vi "界面UI.vi"() -> ()   [LabVIEW 2016, in "科盛超标留样.lvlib"]
uses:
  <vilib>/Utility/miscctls.llb/LVPointTypeDef.ctl
  <vilib>/Utility/config.llb/NI_LVConfig.lvlib
  <vilib>/ptbypt/NI_PtbyPt.lvlib
panel:
  in  "参数设置":bool
  out "留样模式":T1(ring)
  out "仪器时间":timestamp format="%<%Y/%m/%d %H:%M:%S>T"
  out "采样器状态":enum16{"待机", "运行中"}(ring)
  in  "停止流程":bool
  in  "启动流程":bool
  out "流程中":bool
  out "留样等待时间/s":dbl
  out "供样等待时间/s":dbl
  out "采样等待时间/s":dbl
  out "留样完成":bool
  out "采样完成":bool
  out "开关量3状态":T2
  out "开关量2状态":T3
  out "开关量1状态":T4
  out "供样完成":bool
  in  "返回":bool
  in  "查看记录":bool
  out "查询系统状态":T5
  in  "留样命令":bool
  in  "供样命令":bool
  in  "触发采样":bool
  in  "远程取样":bool
  in  "复位指令":bool
  out "VISA resource name":refnum<visa-resource-name>="COM2" caption="VISA资源名称"
  out "读取缓冲区":string
  out "source":string
  out "通讯":bool
  # "启动顺序：\n①先触发采样将水样取到A、B桶\n②然后仪器开始测试时发送供样命令此时供应到分析仪\n③如果超标发送留样命令，如果在默认60分钟(可设置)后都没有接受到超标留\n样指令则自动排空。按不同的采样方式发送不同的通信字符串。在一次采样未结束前不要发送下一个采样指令。"
  # "采样：将水样取到A、B桶的过程；\n供样：将水样从A、B桶供应到分析仪的过程；\n留样：将水样从A、B桶保存到采样瓶的过程。"
  # "科盛超标留样"
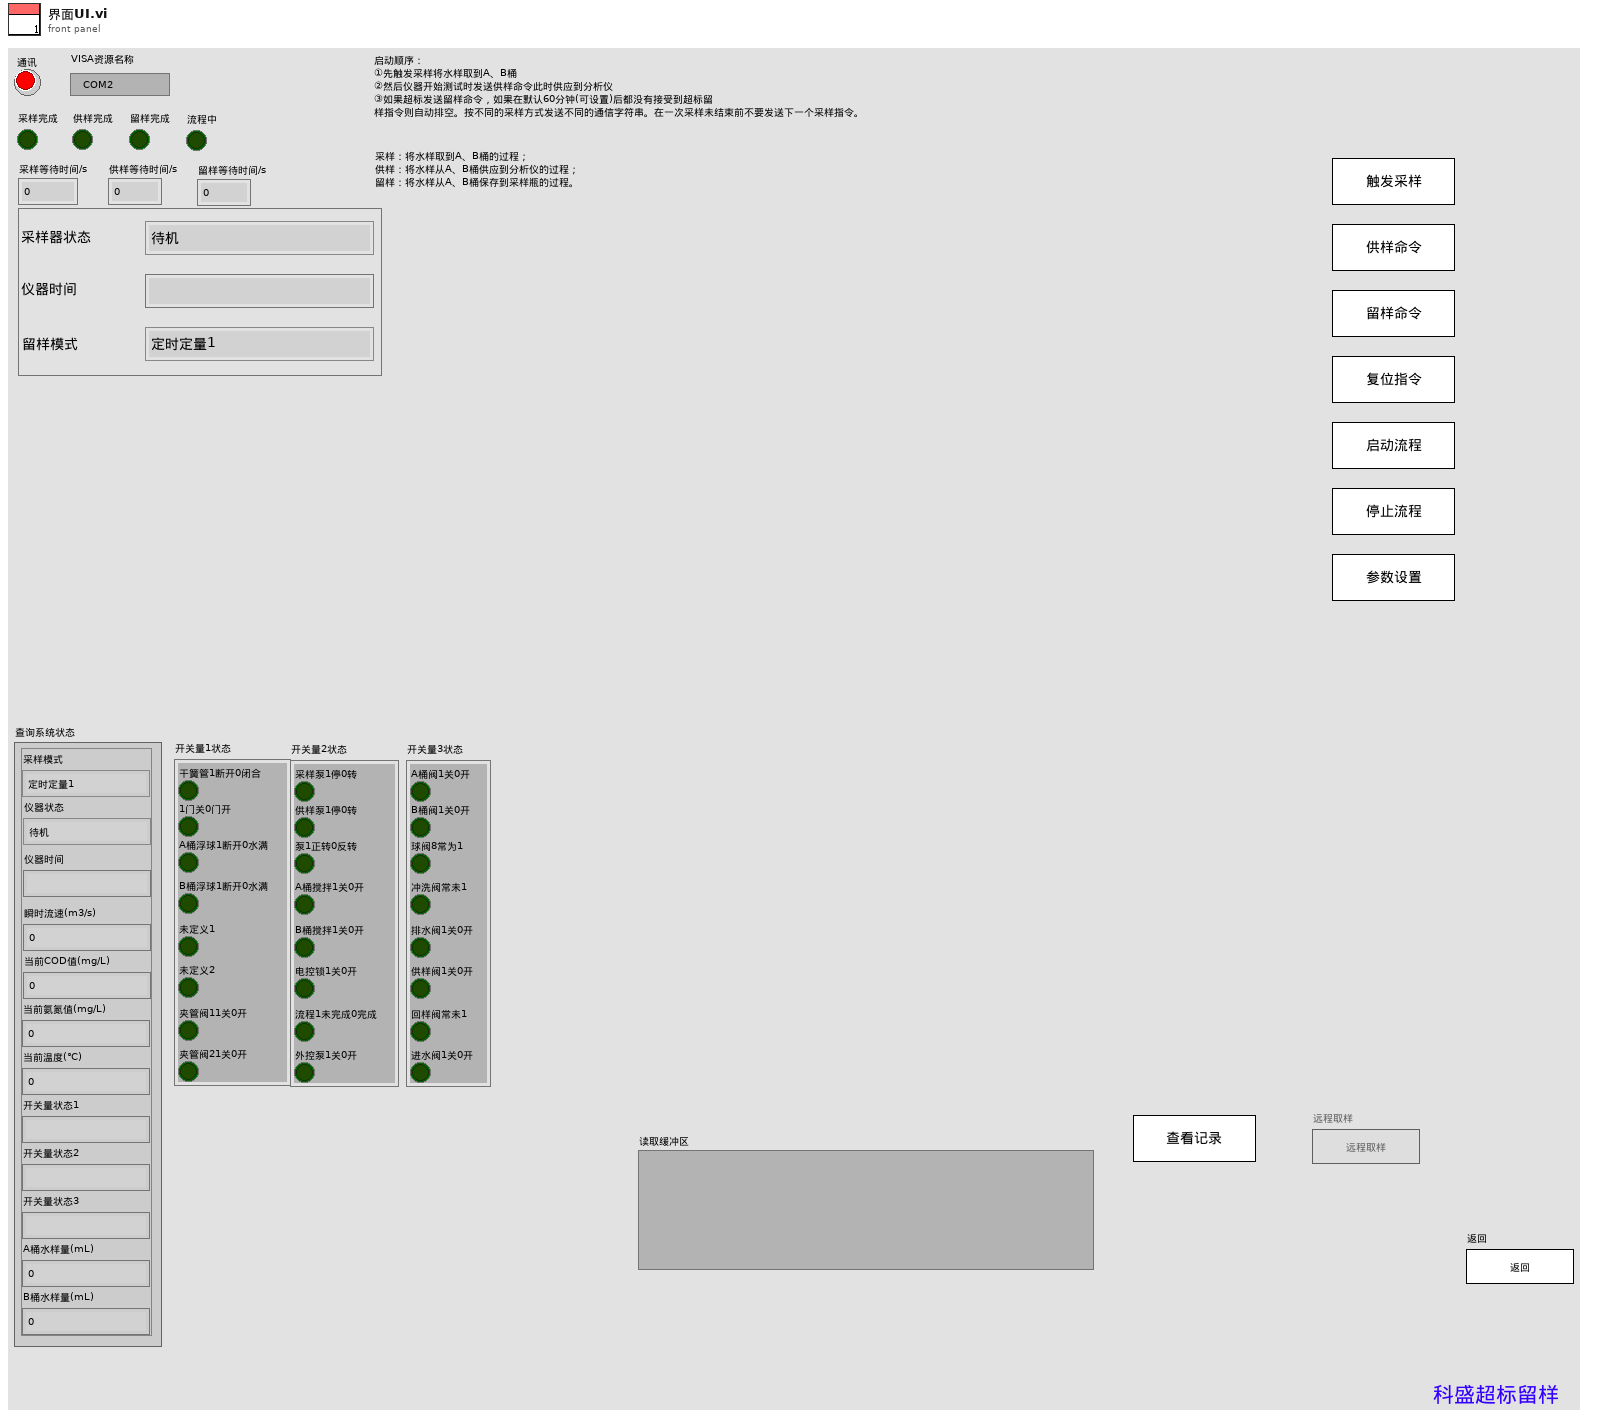
[diagram p1: front panel]
types:
  T1 = enum16{"定时定量1", "定时定量2", "定流定量", "定时比例", "同步留样", "超标留样", "触发采样", "定时采样1", "定流供样", "定时采样2", "远程取样", "手动取样", "流量跟踪"}
  T2 = cluster{"A桶阀1关0开":bool, "B桶阀1关0开":bool, "球阀8常为1":bool, "冲洗阀常未1":bool, "排水阀1关0开":bool, "供样阀1关0开":bool, "回样阀常未1":bool, "进水阀1关0开":bool}
  T3 = cluster{"采样泵1停0转":bool, "供样泵1停0转":bool, "泵1正转0反转":bool, "A桶搅拌1关0开":bool, "B桶搅拌1关0开":bool, "电控锁1关0开":bool, "流程1未完成0完成":bool, "外控泵1关0开":bool}
  T4 = cluster{"干簧管1断开0闭合":bool, "1门关0门开":bool, "A桶浮球1断开0水满":bool, "B桶浮球1断开0水满":bool, "未定义1":bool, "未定义2":bool, "夹管阀11关0开":bool, "夹管阀21关0开":bool}
  T5 = cluster{"采样模式":enum16{"定时定量1", "定时定量2", "定流定量", "定时比例", "同步留样", "超标留样", "触发采样", "定时采样1", "定流供样", "定时采样2", "远程取样", "手动取样", "流量跟踪"}, "仪器状态":enum16{"待机", "运行中"}, "仪器时间":string, "瞬时流速(m3/s)":dbl, "当前COD值(mg/L)":dbl, "当前氨氮值(mg/L)":dbl, "当前温度(℃)":dbl, "开关量状态1":string, "开关量状态2":string, "开关量状态3":string, "A桶水样量(mL)":dbl, "B桶水样量(mL)":dbl}
  T6 = cluster{"枚举":enum16{"open", "read", "write", "close"}, "写入字符串":string, "解析字符串":string}
  T7 = cluster{"STEP":enum16{"open", "read", "write", "close"}, "写入缓冲区":string}
  T8 = enum16{"触发采样", "供样命令", "留样命令", "远程取样", "复位指令", "查询采样记录", "查询瓶记录", "查询系统状态"}
  T9 = typedef "LVPointTypeDef.ctl" = cluster{"Horizontal":i16, "Vertical":i16}
  T10 = typedef "NI_LVConfig.lvlib/Config Data RefNum.ctl" = refnum<k1>
  T11 = enum32{"Bad", "Idle", "Run top level", "Running"}
  T12 = cluster{"命令":string, "data":cluster{"starting address":u16, "coil values":bool[]}}
  T13 = enum8{"Enabled", "Disabled", "Disabled and Grayed Out"}
  T14 = cluster{"[0]":bool, "[1]":bool, "[2]":bool, "[3]":bool, "[4]":bool, "[5]":bool, "[6]":bool, "[7]":bool}
  T15 = cluster{"采样时间":string, "采样模式":enum16{"定时定量1", "定时定量2", "定流定量", "定时比例", "同步留样", "超标留样", "触发采样", "定时采样1", "定流供样", "定时采样2", "远程取样", "手动取样", "流量跟踪"}, "采样瓶":string, "混采n次，设定混采n次":string, "当前采样量(ml)":dbl, "当前瓶内总水样量(ml)":dbl, "当前瓶号平行样，设定平行样":string}[]
  T16 = cluster{"瓶1采样量(ml)":dbl, "瓶2采样量(ml)":dbl, "瓶3采样量(ml)":dbl, "瓶4采样量(ml)":dbl, "瓶5采样量(ml)":dbl, "瓶6采样量(ml)":dbl, "瓶7采样量(ml)":dbl, "瓶8采样量(ml)":dbl, "瓶9采样量(ml)":dbl, "瓶10采样量(ml)":dbl, "瓶11采样量(ml)":dbl, "瓶12采样量(ml)":dbl, "瓶13采样量(ml)":dbl, "瓶14采样量(ml)":dbl, "瓶15采样量(ml)":dbl, "瓶16采样量(ml)":dbl, "瓶17采样量(ml)":dbl, "瓶18采样量(ml)":dbl, "瓶19采样量(ml)":dbl, "瓶20采样量(ml)":dbl, "瓶21采样量(ml)":dbl, "瓶22采样量(ml)":dbl, "瓶23采样量(ml)":dbl, "瓶24采样量(ml)":dbl}
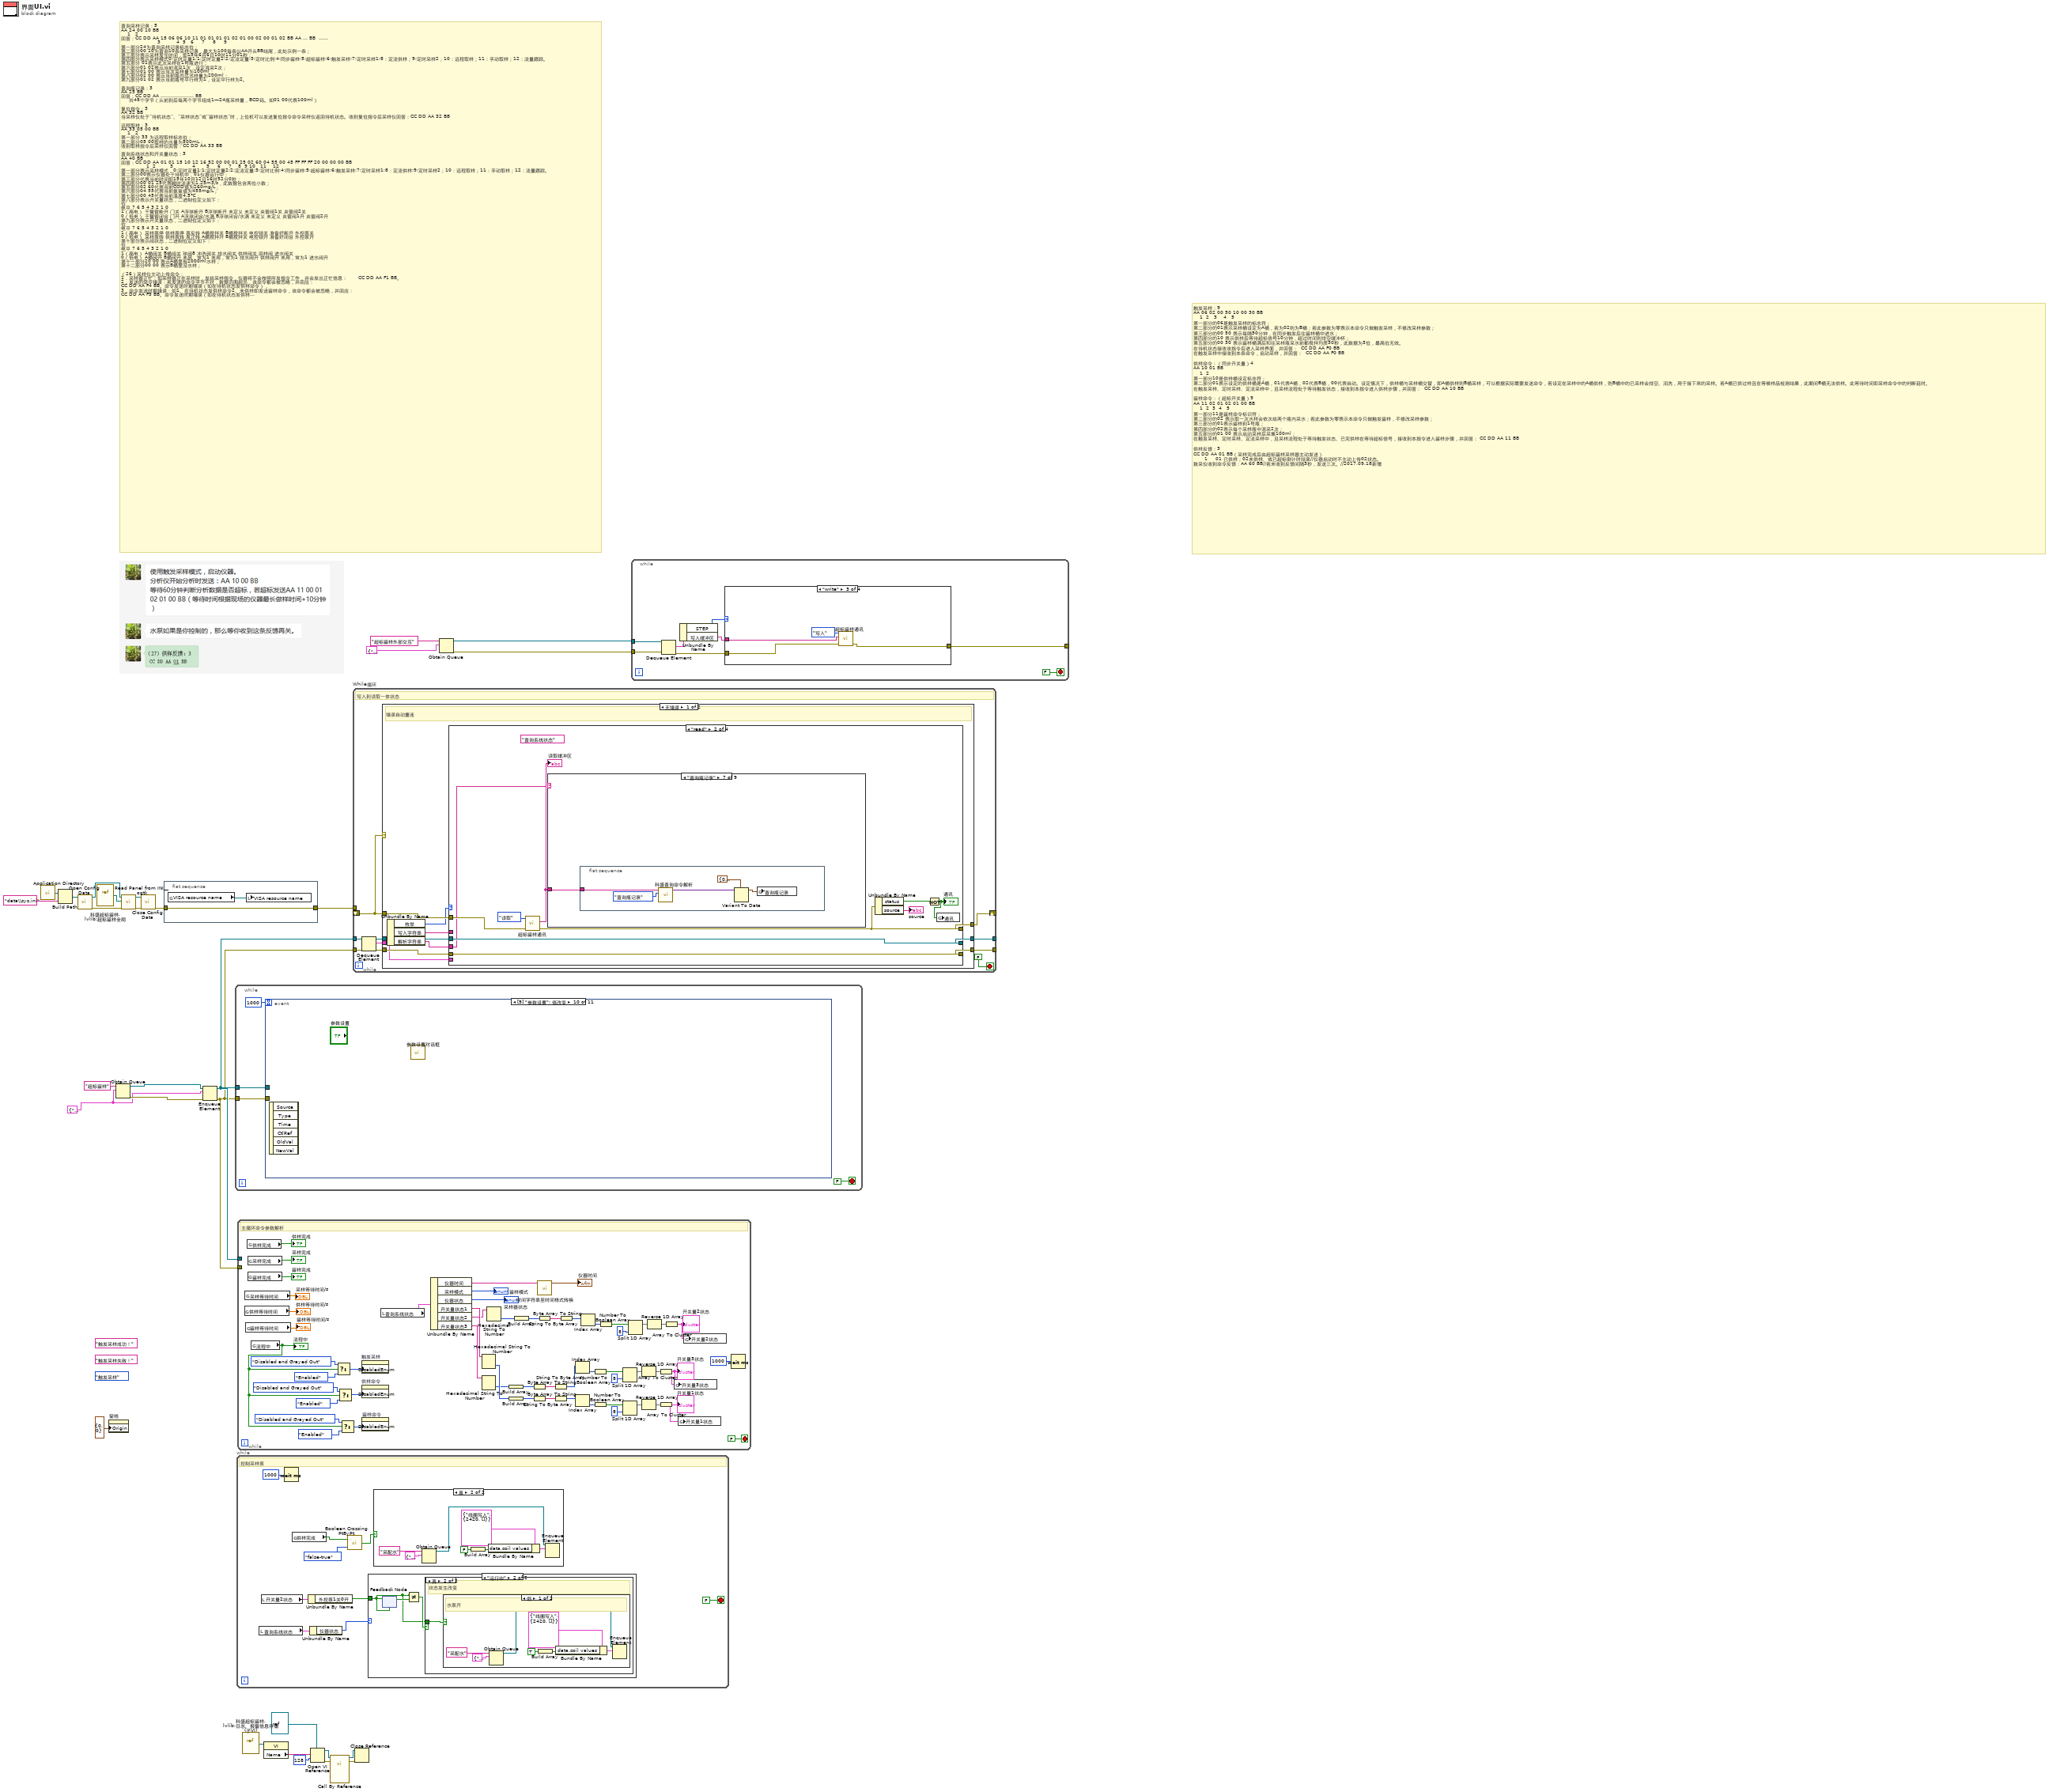
[diagram p0: block diagram]
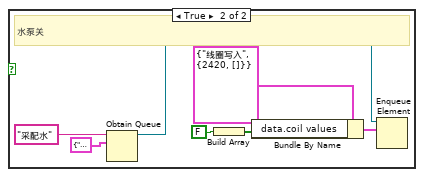
[diagram p4: hidden frame]
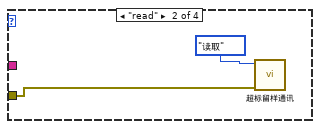
[diagram p7: hidden frame]
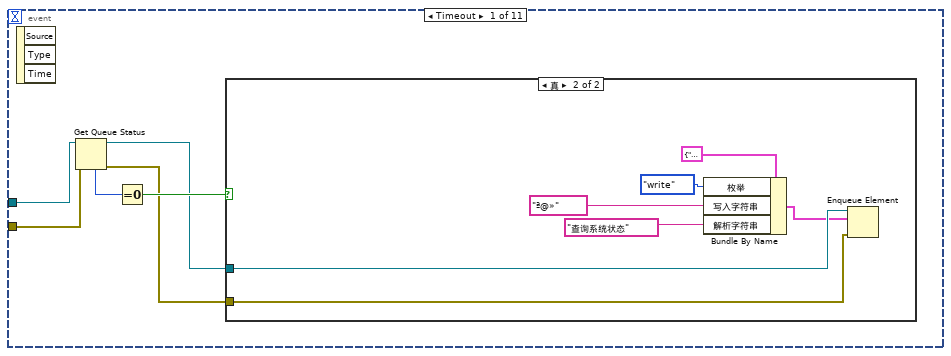
[diagram p9: hidden frame]
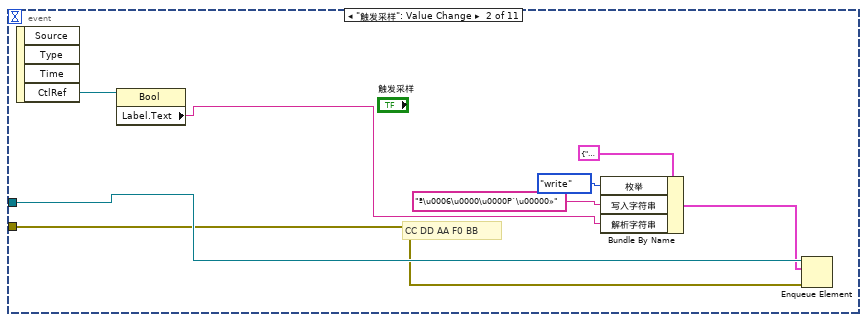
[diagram p11: hidden frame]
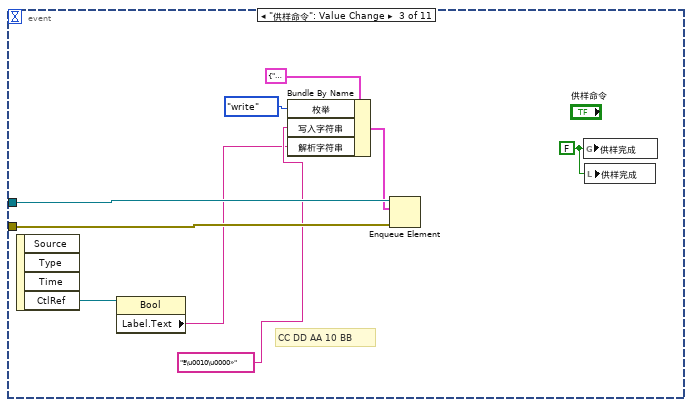
[diagram p12: hidden frame]
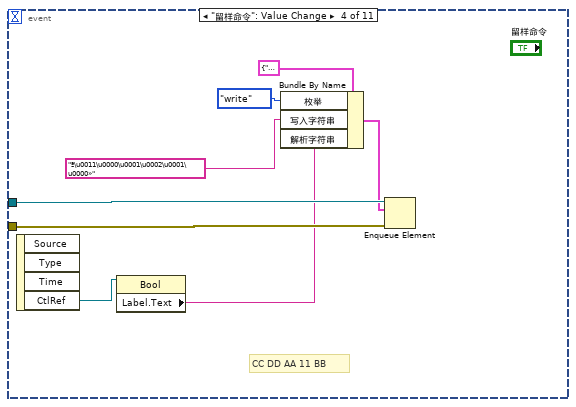
[diagram p13: hidden frame]
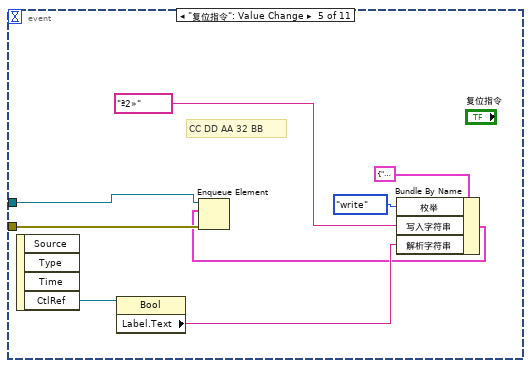
[diagram p14: hidden frame]
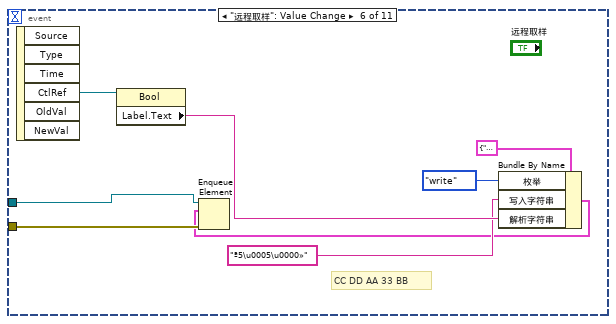
[diagram p15: hidden frame]
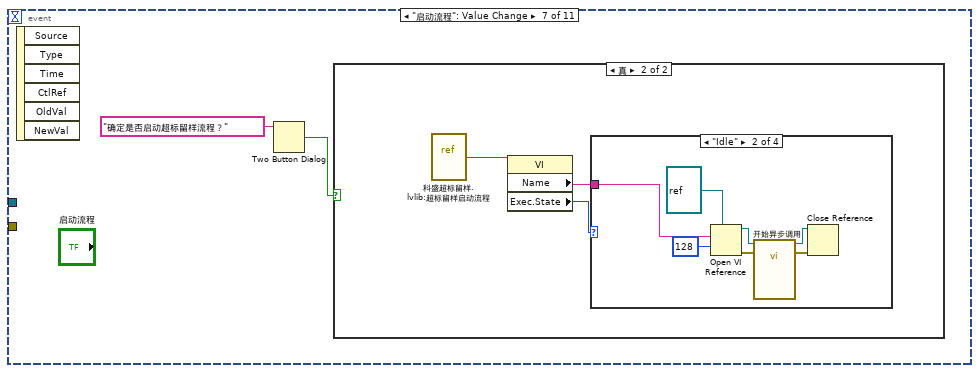
[diagram p16: hidden frame]
diagram:
  w1 = T6 {"枚举"=enum."open", "写入字符串"="", "解析字符串"=""}
  (unwired) "触发采样成功！" ("消息")
  (unwired) "触发采样失败！" ("消息")
  (unwired) T8."触发采样" ("功能输入")
  # "查询采样记录：5\nAA 24 00 10 BB\n    1   2\n回答：CC DD AA 15 06 06 10 11 01 01 01 01 02 01 00 02 00 01 02 BB AA ... BB  ......\n                       3          4  5   6     7     8     9\n第一部分24为查询采样记录标志位；\n第二部分00 10为查询10条采样记录，最大为100每条以AA开头BB结尾，此处示例一条；\n第三部分表示采样发生时间，即15年6月6日10时11分01秒；\n第四部分表示采样模式0:定时定量1;1:定时定量2;2:定流定量;3:定时比例;4:同步留样;5:超标留样;6:触发采样;7:定时采样1;8：定流供样；9:定时采样2；10：远程取样；11：手动取样；12：流量跟踪。\n第五部分 01表示此次采样在1号瓶进行；\n第六部分01 02表示当前混采1次，设定混采2次；\n第七部分01 00 表示当次采样量为100ml；\n第八部分02 00 表示当前瓶内总水样量为200ml；\n第九部分01 02 表示当前瓶号平行样为1，设定平行样为2。\n\n查询瓶记录：3\nAA 25 BB\n回答：CC DD AA ………………… BB\n     共48个字节（从前到后每两个字节组成1—24瓶采样量，BCD码。如01 00代表100ml）\n\n复位指令：3\nAA 32 BB\n当采样仪处于“待机状态”、“采样状态”或“留样状态”时，上位机可以发送复位指令命令采样仪返回待机状态。收到复位指令后采样仪回答：CC DD AA 32 BB\n\n远程取样：3\nAA 33 05 00 BB\n    1   2\n第一部分 33 为远程取样标志位；\n第二部分05 00取样的水量为500mL；\n收到取样指令后采样仪回答：CC DD AA 33 BB\n\n查询系统状态和开关量状态：3\nAA 40 BB\n回答：CC DD AA 01 01 15 10 12 16 52 00 00 01 25 02 60 04 55 00 45 FF FF FF 20 00 00 00 BB \n                1  2         3            4       5     6     7    8  9 10   11    12  \n第一部分表示采样模式，0:定时定量1;1:定时定量2;2:定流定量;3:定时比例;4:同步留样;5:超标留样;6:触发采样;7:定时采样1;8：定流供样;9:定时采样2；10：远程取样；11：手动取样；12：流量跟踪。\n第二部分00表示仪器处于待机中，01仪器运行中；\n第三部分代表当前时间即15年10月12日16时52分0秒； \n第四部分00 01 25代表瞬时流速为1.25m3/s，此数据包含两位小数；\n第五部分02 60代表当前COD值为260mg/L；\n第六部分04 55代表当前氨氮值为455mg/L；\n第七部分00 45代表当前温度4.5℃；\n第八部分表示开关量状态，二进制位定义如下：\n位\n电平\t7\t6\t5\t4\t3\t2\t1\t0\n1（高电）\t干簧管断开\t门关\tA浮球断开\tB浮球断开\t未定义\t未定义\t夹管阀1关\t夹管阀2关\n0（低电）\t干簧管闭合\t门开\tA浮球闭合/水满\tB浮球闭合/水满\t未定义\t未定义\t夹管阀1开\t夹管阀2开\n第九部分表示开关量状态，二进制位定义如下：\n位\n电平\t7\t6\t5\t4\t3\t2\t1\t0\n1（高电）\t采样泵停\t供样泵停\t泵反转\tA桶搅拌关\tB桶搅拌关\t电控锁关\t准备好断开\t外控泵关\n0（低电）\t采样泵转\t供样泵转\t泵正转\tA桶搅拌开\tB桶搅拌关\t电控锁开\t准备好闭合\t外控泵开\n第十部分表示阀状态，二进制位定义如下：\n位\n电平\t7\t6\t5\t4\t3\t2\t1\t0\n1（高电）\tA桶阀关\tB桶阀关\t球阀8\t冲洗阀关\t排水阀关\t供样阀关\t回样阀\t进水阀关\n0（低电）\tA桶阀开\tB桶阀开\t未用，常为1\t未用，常为1\t排水阀开\t供样阀开\t未用，常为1\t进水阀开\n第十一部分20 00 表示A桶里有2000ml水样；\n第十二部分00 00 表示B桶里没水样；\n\n（26）采样仪主动上传命令：\n1．采样器正忙：如采样器正在采样时，发给采样指令，仪器将不会按照所发指令工作，并会发出正忙信息：\t\t     CC DD AA F1 BB。\n2．发送的命令错误：若发送的命令字节不对，数据范围超出，该命令都会被忽略，并回应：\nCC DD AA F4 BB。命令发送时期错误（如在待机状态发供样命令），\n3．命令发送时期错误：如1、在待机状态发供样命令2、未供样即发送留样命令，该命令都会被忽略，并回应：\nCC DD AA F5 BB。命令发送时期错误（如在待机状态发供样命令），\n \t4．系统切换进入忙状态：仪器主动上传CC DD AA F6 BB。\n5．系统切换进入空闲状态：仪器主动上传CC DD AA F7 BB。"
  # "触发采样：9\nAA 06 02 00 50 10 00 30 BB\n    1  2   3    4   5         \n第一部分的06是触发采样的标志符；\n第二部分的01表示采样桶设定为A桶，若为02则为B桶；若此参数为零表示本命令只做触发采样，不修改采样参数；\n第三部分的00 50 表示每隔50分钟，在同步触发后往留样桶中进水；\n第四部分的10 表示供样后等待超标信号10分钟，超过时间则排空缓冲杯；\n第五部分的00 30 表示留样桶满后和往采样瓶采水前都搅拌均质30秒，此数据为3位，最高位无效。\n在待机状态接收该指令后进入采样界面，并回答：\t\tCC DD AA F0 BB\n在触发采样中接收到本条命令，启动采样，并回答：\t\tCC DD AA F0 BB\n\n供样命令：（同步开关量）4\nAA 10 01 BB\n    1  2  \n第一部分10是供样桶设定标志符；\n第二部分01表示设定的供样桶是A桶，01代表A桶，02代表B桶，00代表自动。设定情况下，供样桶与采样桶交替，即A桶供样则B桶采样，可以根据实际需要发送命令，若设定在采样中的A桶供样，则B桶中的已采样会排空、润洗，用于接下来的采样。若A桶已供过样且在等候样品检测结果，此期间B桶无法供样。此等待时间即采样命令中的判断延时。\n在触发采样、定时采样、定流采样中，且采样流程处于等待触发状态，接收到本指令进入供样步骤，并回答：\t\tCC DD AA 10 BB\n\n留样命令：（超标开关量）9\nAA 11 02 01 02 01 00 BB\n    1  2  3  4   5    \n第一部分11是留样命令标识符；\n第二部分的02 表示取一次水样会依次给两个瓶内采水；若此参数为零表示本命令只做触发留样，不修改采样参数；\n第三部分的01表示留样到1号瓶；\n第四部分的02表示每个采样瓶中混采2次；\n第五部分的01 00 表示启动采样后采集100ml；\n在触发采样、定时采样、定流采样中，且采样流程处于等待触发状态、已完供样在等待超标信号，接收到本指令进入留样步骤，并回答：\tCC DD AA 11 BB\n\n供样反馈：3\nCC DD AA 01 BB（采样完成后由超标留样采样器主动发送）\n  \t\t   1  \t\t\t01 已供样；02未供样、或已超标倒计时结束//仪器启动时不主动上传02状态。\n数采仪收到命令反馈：AA 60 BB//若未收到反馈间隔3秒，发送三次。//2017.09.18新增"
  n1 = call <vilib>:"Application Directory.vi"() -> ("Application Directory"=w23:path)
  n2 = Build Path(base path=w23, name or relative path="data\\sys.ini" ("名称或相对路径")) -> (appended path=w21:path)
  n3 = call <vilib>:"Open Config Data.vi"("configuration file path"=w21) -> ("error out"=w17:errorcluster, "refnum"=w20:T10)  [unwired: 8 in, 1 out]
  n4 = vi-ref "科盛超标留样.lvlib:超标留样全局.vi"() -> (w19:refnum<vi>)
  n5 = property on="窗格" class="Pane"("Origin"=T9 {"Horizontal"=0, "Vertical"=0} ("原点")) -> ()  [unwired: 2 in, 2 out]
  n6 = Obtain Queue(name (unnamed)="超标留样" ("名称（未命名）"), element data type=w1) -> (queue out=w28:refnum<queue>, error out=w27:errorcluster)  [unwired: 3 in, 1 out]
  n7 = call <userlib>:"Read Panel from INI__ogtk.vi"("error in (no error)"=w17, "VI ref"=w19, "refnum"=w20) -> ("error out"=w16:errorcluster, "refnum out"=w18:T10)  [unwired: 7 in]
  n8 = call <vilib>:"Close Config Data.vi"("error in (no error)"=w16, "refnum"=w18) -> ("error out"=w15:errorcluster)  [unwired: 8 in, 1 out]
  n9 = flat-sequence {
    tunnel: w15 -> [w30]
    tunnel: [w30] -> w14
    frame #0 {
      n10 = global read "超标留样全局.vi" "VISA resource name"() -> (w31:refnum<visa-resource-name>)
      n11 = local write "VISA resource name"(w31) -> ()
    }
  }
  n12 = Enqueue Element(queue=w28, element=w1, error in (no error)=w27) -> (queue out=w26:refnum<queue>, error out=w25:errorcluster)  [unwired: 1 in, 1 out]
  n13 = while {
    tunnel: w26 -> [w34]
    tunnel: w25 -> [w33]
    stop <- FALSE stop-if-true
    n14 = event shown="[9] \"参数设置\": 值改变" {
      selector: _ -> [_ _ _ _ _ _ _ _ _ _ _]
      dyn-events: _ -> [_ _ _ _ _ _ _ _ _ _ _]
      timeout: 1000 -> [_ _ _ _ _ _ _ _ _ _ _]
      tunnel: w34 -> [w40 w56 w64 w73 w81 w89 _ w103 _ _ _]
      tunnel: w33 -> [w39 w55 w65 w72 w80 w88 _ w102 _ _ _]
      event Timeout {
        n15 = event-data() -> ()  [unwired: 1 in, 3 out]
        n16 = Get Queue Status(queue=w40, error in (no error)=w39) -> (queue out=w37:refnum<queue>, error out=w36:errorcluster, # elements in queue=w41:i32)  [unwired: 1 in, 5 out]
        n17 = Equal To 0?(x=w41) -> (x = 0?=w38:bool)
        n18 = case shown="真" w38 {
          tunnel: w37 -> [_ w48]
          tunnel: w36 -> [_ w47]
          frame False {
          }
          frame True {
            n19 = Bundle By Name(cluster=T6 {"枚举"=enum."open", "写入字符串"="", "解析字符串"=""}, "枚举"=enum16{"open", "read", "write", "close"}."write" ("元素"), "写入字符串"="ª@»" ("写入缓冲区"), "解析字符串"="查询系统状态" ("当前解析模式")) -> (w42:T6)
            n20 = Enqueue Element(queue=w48, element=w42, error in (no error)=w47) -> ()  [unwired: 1 in, 3 out]
          }
        }
      }
      event "触发采样": Value Change {
        # "CC DD AA F0 BB"
        n21 = event-data() -> ("CtlRef"=w54:refnum<vi>)  [unwired: 1 in, 3 out]
        n22 = property class="Bool"(reference=w54) -> ("Label.Text"=w50:string)  [unwired: 1 in, 2 out]
        n23 = Bundle By Name(cluster=T6 {"枚举"=enum."open", "写入字符串"="", "解析字符串"=""}, "枚举"=enum16{"open", "read", "write", "close"}."write" ("元素"), "写入字符串"="ª\u0006\u0000\u0000P`\u00000»" ("写入缓冲区"), "解析字符串"=w50) -> (w49:T6)
        n24 = Enqueue Element(queue=w56, element=w49, error in (no error)=w55) -> ()  [unwired: 1 in, 3 out]
      }
      event "供样命令": Value Change {
        w62 = FALSE ("供样完成")
        # "CC DD AA 10 BB"
        n25 = event-data() -> ("CtlRef"=w63:refnum<vi>)  [unwired: 1 in, 3 out]
        n26 = property class="Bool"(reference=w63) -> ("Label.Text"=w58:string)  [unwired: 1 in, 2 out]
        n27 = Bundle By Name(cluster=T6 {"枚举"=enum."open", "写入字符串"="", "解析字符串"=""}, "枚举"=enum16{"open", "read", "write", "close"}."write" ("元素"), "写入字符串"="ª\u0010\u0000»" ("写入缓冲区"), "解析字符串"=w58) -> (w57:T6)
        n28 = Enqueue Element(queue=w64, element=w57, error in (no error)=w65) -> ()  [unwired: 1 in, 3 out]
        n29 = global write "超标留样全局.vi" "供样完成"(w62) -> ()
        n30 = local write "供样完成"(w62) -> ()
      }
      event "留样命令": Value Change {
        # "CC DD AA 11 BB"
        n31 = event-data() -> ("CtlRef"=w71:refnum<vi>)  [unwired: 1 in, 3 out]
        n32 = property class="Bool"(reference=w71) -> ("Label.Text"=w67:string)  [unwired: 1 in, 2 out]
        n33 = Bundle By Name(cluster=T6 {"枚举"=enum."open", "写入字符串"="", "解析字符串"=""}, "枚举"=enum16{"open", "read", "write", "close"}."write" ("元素"), "写入字符串"="ª\u0011\u0000\u0001\u0002\u0001\u0000»" ("写入缓冲区"), "解析字符串"=w67) -> (w66:T6)
        n34 = Enqueue Element(queue=w73, element=w66, error in (no error)=w72) -> ()  [unwired: 1 in, 3 out]
      }
      event "复位指令": Value Change {
        # "CC DD AA 32 BB"
        n35 = event-data() -> ("CtlRef"=w79:refnum<vi>)  [unwired: 1 in, 3 out]
        n36 = property class="Bool"(reference=w79) -> ("Label.Text"=w75:string)  [unwired: 1 in, 2 out]
        n37 = Bundle By Name(cluster=T6 {"枚举"=enum."open", "写入字符串"="", "解析字符串"=""}, "枚举"=enum16{"open", "read", "write", "close"}."write" ("元素"), "写入字符串"="ª2»" ("写入缓冲区"), "解析字符串"=w75) -> (w74:T6)
        n38 = Enqueue Element(queue=w81, element=w74, error in (no error)=w80) -> ()  [unwired: 1 in, 3 out]
      }
      event "远程取样": Value Change {
        # "CC DD AA 33 BB"
        n39 = event-data() -> ("CtlRef"=w87:refnum<vi>)  [unwired: 1 in, 5 out]
        n40 = property class="Bool"(reference=w87) -> ("Label.Text"=w84:string)  [unwired: 1 in, 2 out]
        n41 = Bundle By Name(cluster=T6 {"枚举"=enum."open", "写入字符串"="", "解析字符串"=""}, "枚举"=enum16{"open", "read", "write", "close"}."write" ("元素"), "写入字符串"="ª5\u0005\u0000»" ("写入缓冲区"), "解析字符串"=w84) -> (w82:T6)
        n42 = Enqueue Element(queue=w89, element=w82, error in (no error)=w88) -> ()  [unwired: 1 in, 3 out]
      }
      event "启动流程": Value Change {
        n43 = event-data() -> ()  [unwired: 1 in, 6 out]
        n44 = Two Button Dialog(message="确定是否启动超标留样流程？" ("消息")) -> (T button?=w90:bool)  [unwired: 2 in]
        n45 = case shown="真" w90 {
          frame False {
          }
          frame True {
            n46 = vi-ref "科盛超标留样.lvlib:超标留样启动流程.vi"() -> (w92:refnum<vi>)
            n47 = property class="VI"(reference=w92) -> ("Name"=w93:string, "Exec.State"=w94:T11)  [unwired: 1 in, 2 out]
            n48 = case shown="\"Idle\"" w94 {
              tunnel: w93 -> [_ w97 _ _]
              frame "Bad", Default {
              }
              frame "Idle" {
                n49 = Open VI Reference(type specifier VI Refnum (for type only)=refnum<vi> refnum ("类型说明符VI引用句柄（仅用于类型）"), vi path=w97, options=128 ("选项")) -> (vi reference=w101:refnum<vi>, error out=w96:errorcluster)  [unwired: 3 in]
                n50 = call-by-ref "开始异步调用"(reference=w101, error in=w96) -> (reference out=w100:refnum<vi>, error out=w95:errorcluster)  [unwired: 12 in]
                n51 = Close Reference(reference=w100, error in (no error)=w95) -> ()  [unwired: 1 out]
              }
              frame "Run top level" {
              }
              frame "Running" {
              }
            }
          }
        }
      }
      event "停止流程": Value Change {
        n52 = event-data() -> ()  [unwired: 1 in, 6 out]
        n53 = Two Button Dialog(message="确定是否停止超标留样流程？" ("消息")) -> (T button?=w104:bool)  [unwired: 2 in]
        n54 = case shown="真" w104 {
          tunnel: w103 -> [_ w111]
          tunnel: w102 -> [_ w110]
          frame False {
          }
          frame True {
            n55 = Obtain Notifier(name (unnamed)="超标留样流程" ("名称（未命名）"), notification data type=FALSE ("采样完成")) -> (notifier out=w116:refnum<notifier>, error out=w115:errorcluster)  [unwired: 2 in, 1 out]
            n56 = Send Notification(notification=TRUE ("通知"), notifier=w116, error in (no error)=w115) -> (notifier out=w113:refnum<notifier>, error out=w112:errorcluster)
            n57 = Release Notifier(notifier=w113, error in (no error)=w112) -> ()  [unwired: 1 in, 3 out]
            n58 = Bundle By Name(cluster=T6 {"枚举"=enum."open", "写入字符串"="", "解析字符串"=""}, "枚举"=enum16{"open", "read", "write", "close"}."write" ("元素"), "写入字符串"="ª2»" ("写入缓冲区")) -> (w106:T6)
            n59 = Enqueue Element(queue=w111, element=w106, error in (no error)=w110) -> ()  [unwired: 1 in, 3 out]
          }
        }
      }
      event "查看记录": Value Change {
        n60 = event-data() -> ()  [unwired: 1 in, 6 out]
        n61 = property on="窗格" class="Pane"("Origin"=T9 {"Horizontal"=0, "Vertical"=628} ("原点")) -> ()  [unwired: 2 in, 2 out]
      }
      event "参数设置": Value Change {
        n62 = event-data() -> ()  [unwired: 1 in, 6 out]
        n63 = call "参数设置对话框.vi"() -> ()  [unwired: 12 in]
      }
      event "返回": Value Change {
        n64 = event-data() -> ()  [unwired: 1 in, 6 out]
        n65 = property on="窗格" class="Pane"("Origin"=T9 {"Horizontal"=0, "Vertical"=0} ("原点")) -> ()  [unwired: 2 in, 2 out]
      }
    }
  }
  n66 = while {
    stop <- FALSE stop-if-true
    # "控制采样泵"
    n67 = local read "查询系统状态"() -> (w123:T5)
    n68 = local read "开关量2状态"() -> (w124:T3)
    n69 = Wait (ms)(milliseconds to wait=u32 1000 ("等待时间（毫秒）")) -> ()  [unwired: 1 out]
    n70 = global read "超标留样全局.vi" "供样完成"() -> (w126:bool)
    n71 = Unbundle By Name(w124) -> ("外控泵1关0开"=w121:bool)
    n72 = Unbundle By Name(w123) -> ("仪器状态"=w122:enum16{"待机", "运行中"})
    n73 = call <vilib>:"Boolean Crossing PtByPt.vi"("direction"=enum16{"either", "false-true", "true-false"}."false-true", "input"=w126) -> ("crossing"=w125:bool)  [unwired: 1 in]
    n74 = case shown="\"运行中\"" w122 {
      tunnel: w121 -> [_ w130]
      frame "待机", Default {
      }
      frame "运行中" {
        n75 = feedback-in #1(w130) -> ()
        n76 = feedback #1(w130) -> (w132:bool)
        n77 = Not Equal?(x=w130, y=w132) -> (x != y?=w131:bool)
        n78 = case shown="真" w131 {
          tunnel: w130 -> [_ w133]
          frame False {
          }
          frame True {
            # "状态发生改变"
            n79 = case shown="假" w133 {
              frame False {
                # "水泵开"
                n80 = Obtain Queue(name (unnamed)="采配水" ("名称（未命名）"), element data type=cluster{"命令":string, "数据":variant} {"命令"="", "数据"=variant}) -> (queue out=w134:refnum<queue>)  [unwired: 3 in, 2 out]
                n81 = Build Array(TRUE) -> (w137:bool[])
                n82 = Bundle By Name(cluster=T12 {"命令"="线圈写入", "data"={"starting address"=2420, "coil values"=[]}} ("元素"), "data.coil values"=w137) -> (w139:T12)
                n83 = Enqueue Element(queue=w134, element=w139) -> ()  [unwired: 2 in, 3 out]
              }
              frame True {
                # "水泵关"
                n84 = Obtain Queue(name (unnamed)="采配水" ("名称（未命名）"), element data type=cluster{"命令":string, "数据":variant} {"命令"="", "数据"=variant}) -> (queue out=w141:refnum<queue>)  [unwired: 3 in, 2 out]
                n85 = Build Array(FALSE) -> (w144:bool[])
                n86 = Bundle By Name(cluster=T12 {"命令"="线圈写入", "data"={"starting address"=2420, "coil values"=[]}} ("元素"), "data.coil values"=w144) -> (w146:T12)
                n87 = Enqueue Element(queue=w141, element=w146) -> ()  [unwired: 2 in, 3 out]
              }
            }
          }
        }
      }
    }
    n88 = case shown="真" w125 {
      frame False {
      }
      frame True {
        n89 = Obtain Queue(name (unnamed)="采配水" ("名称（未命名）"), element data type=cluster{"命令":string, "数据":variant} {"命令"="", "数据"=variant}) -> (queue out=w148:refnum<queue>)  [unwired: 3 in, 2 out]
        n90 = Build Array(FALSE) -> (w151:bool[])
        n91 = Bundle By Name(cluster=T12 {"命令"="线圈写入", "data"={"starting address"=2420, "coil values"=[]}} ("元素"), "data.coil values"=w151) -> (w153:T12)
        n92 = Enqueue Element(queue=w148, element=w153) -> ()  [unwired: 2 in, 3 out]
      }
    }
  }
  n93 = while {
    tunnel: w26 -> [_]
    tunnel: w25 -> [_]
    stop <- FALSE stop-if-true
    # "主循环命令参数解析"
    n94 = global read "超标留样全局.vi" "供样等待时间"() -> (→"供样等待时间/s":dbl)
    n95 = global read "超标留样全局.vi" "采样等待时间"() -> (→"采样等待时间/s":dbl)
    n96 = global read "超标留样全局.vi" "留样等待时间"() -> (→"留样等待时间/s":dbl)
    n97 = global read "超标留样全局.vi" "供样完成"() -> (→"供样完成":bool)
    n98 = global read "超标留样全局.vi" "采样完成"() -> (→"采样完成":bool)
    n99 = global read "超标留样全局.vi" "留样完成"() -> (→"留样完成":bool)
    n100 = global read "超标留样全局.vi" "流程中"() -> (w161:bool)
    "流程中" <- w161
    n101 = Select(t=T13."Disabled and Grayed Out" ("禁用"), s=w161, f=T13."Enabled" ("禁用")) -> (s? t:f=w168:T13)
    n102 = Select(t=T13."Disabled and Grayed Out" ("禁用"), s=w161, f=T13."Enabled" ("禁用")) -> (s? t:f=w160:T13)
    n103 = Select(t=T13."Disabled and Grayed Out" ("禁用"), s=w161, f=T13."Enabled" ("禁用")) -> (s? t:f=w159:T13)
    n104 = property on="触发采样" class="Bool"("DisabledEnum"=w168) -> ()  [unwired: 2 in, 2 out]
    n105 = property on="供样命令" class="Bool"("DisabledEnum"=w160) -> ()  [unwired: 2 in, 2 out]
    n106 = property on="留样命令" class="Bool"("DisabledEnum"=w159) -> ()  [unwired: 2 in, 2 out]
    n107 = local read "查询系统状态"() -> (w208:T5)
    n108 = Unbundle By Name(w208) -> ("仪器时间"=w156:string, "采样模式"=→"留样模式":T1, "仪器状态"=→"采样器状态":enum16{"待机", "运行中"}, "开关量状态1"=w183:string, "开关量状态2"=w182:string, "开关量状态3"=w181:string)
    n109 = Hexadecimal String To Number(string=w183) -> (number=w189:u32)  [unwired: 2 in, 1 out]
    n110 = Hexadecimal String To Number(string=w181) -> (number=w185:u32)  [unwired: 2 in, 1 out]
    n111 = Hexadecimal String To Number(string=w182) -> (number=w186:u32)  [unwired: 2 in, 1 out]
    n112 = Build Array(w185) -> (w184:u32[])
    n113 = Build Array(w189) -> (w188:u32[])
    n114 = Build Array(w186) -> (w187:u32[])
    n115 = Byte Array To String(unsigned byte array=w184) -> (string=w178:string)
    n116 = Byte Array To String(unsigned byte array=w188) -> (string=w180:string)
    n117 = call "时间字符串至时间格式转换.vi"("字符串"=w156) -> ("seconds since 1Jan1904"=→"仪器时间":timestamp)  [unwired: 10 in]
    n118 = Byte Array To String(unsigned byte array=w187) -> (string=w179:string)
    n119 = String To Byte Array(string=w178) -> (unsigned byte array=w197:u8[])
    n120 = String To Byte Array(string=w180) -> (unsigned byte array=w207:u8[])
    n121 = String To Byte Array(string=w179) -> (unsigned byte array=w198:u8[])
    n122 = Index Array(array=w197) -> (element=w194:u8)  [unwired: 1 in]
    n123 = Index Array(array=w207) -> (element=w204:u8)  [unwired: 1 in]
    n124 = Index Array(array=w198) -> (element=w201:u8)  [unwired: 1 in]
    n125 = Number To Boolean Array(number=w194) -> (Boolean array=w193:bool[])
    n126 = Number To Boolean Array(number=w204) -> (Boolean array=w203:bool[])
    n127 = Number To Boolean Array(number=w201) -> (Boolean array=w202:bool[])
    n128 = Split 1D Array(array=w193, index=8 ("索引")) -> (first subarray=w196:bool[])  [unwired: 1 out]
    n129 = Split 1D Array(array=w203, index=8 ("索引")) -> (first subarray=w206:bool[])  [unwired: 1 out]
    n130 = Split 1D Array(array=w202, index=8 ("索引")) -> (first subarray=w199:bool[])  [unwired: 1 out]
    n131 = Reverse 1D Array(array=w196) -> (reversed array=w190:bool[])
    n132 = Reverse 1D Array(array=w206) -> (reversed array=w192:bool[])
    n133 = Reverse 1D Array(array=w199) -> (reversed array=w191:bool[])
    n134 = Array To Cluster(array=w190) -> (cluster=w176:T14)
    "开关量3状态" <- w176
    n135 = Array To Cluster(array=w192) -> (cluster=w177:T14)
    "开关量1状态" <- w177
    n136 = Array To Cluster(array=w191) -> (cluster=w175:T14)
    "开关量2状态" <- w175
    n137 = global write "超标留样全局.vi" "开关量3状态"(w176) -> ()
    n138 = global write "超标留样全局.vi" "开关量1状态"(w177) -> ()
    n139 = global write "超标留样全局.vi" "开关量2状态"(w175) -> ()
    n140 = Wait (ms)(milliseconds to wait=u32 1000 ("等待时间（毫秒）")) -> ()  [unwired: 1 out]
  }
  n141 = vi-ref "科盛超标留样.lvlib:日志、报警信息存储 (子VI).vi"() -> (w9:refnum<vi>)
  n142 = property class="VI"(reference=w9) -> ("Name"=w8:string)  [unwired: 1 in, 2 out]
  n143 = Open VI Reference(type specifier VI Refnum (for type only)=refnum<vi> refnum ("类型说明符VI引用句柄（仅用于类型）"), vi path=w8, options=128 ("选项")) -> (vi reference=w5:refnum<vi>, error out=w2:errorcluster)  [unwired: 3 in]
  n144 = call-by-ref "?"(reference=w5, error in=w2) -> (reference out=w4:refnum<vi>, error out=w3:errorcluster)  [unwired: 12 in]
  n145 = while "While循环" {
    tunnel: w26 -> [w219]
    tunnel: w25 -> [w218]
    tunnel: [w214] -> _
    tunnel: [w213] -> _
    shift-right: [w211] -> _
    shift-left: _ -> [w212]
    tunnel: w14 -> [_]
    stop <- FALSE stop-if-true
    # "写入到读取一体状态"
    n146 = Dequeue Element(queue=w219, error in (no error)=w218) -> (queue out=w216:refnum<queue>, element=w217:T6, error out=w215:errorcluster)  [unwired: 1 in, 1 out]
    n147 = case shown="无错误" w212 {
      tunnel: w217 -> [w222 _]
      tunnel: w216 -> [w230 w345]
      tunnel: w215 -> [w229 w344]
      tunnel: [w228 w339] -> w214
      tunnel: [w227 w338] -> w213
      tunnel: w212 -> [w226 w341]
      tunnel: [w225 w340] -> w211
      frame No Error {
        # "错误自动重连"
        n148 = Unbundle By Name(w222) -> ("枚举"=w224:enum16{"open", "read", "write", "close"}, "写入字符串"=w223:string, "解析字符串"=w221:string)
        n149 = case shown="\"read\"" w224 {
          tunnel: [w231 w238 w317 w331] -> w225
          tunnel: w230 -> [w234 w243 w323 w330]
          tunnel: w229 -> [w233 w242 w322 w329]
          tunnel: [w234 w243 w321 w328] -> w228
          tunnel: [w233 w242 w320 w327] -> w227
          tunnel: w226 -> [_ w245 w319 w333]
          tunnel: w223 -> [_ _ w316 _]
          tunnel: w222 -> [_ _ w315 _]
          tunnel: w221 -> [_ w236 w313 _]
          frame "open", Default {
            (unwired) refnum<visa-resource-name> "COM2" ("VISA resource name")
            n150 = global read "超标留样全局.vi" "VISA resource name"() -> (w232:refnum<visa-resource-name>)
            "VISA resource name" <- w232
            n151 = call "超标留样通讯.vi"("VISA resource name"=w232, "功能输入"=enum16{"打开串口", "写入", "读取", "关闭串口"}."打开串口") -> ("error out"=w231:errorcluster)  [unwired: 7 in, 2 out]
          }
          frame "read" {
            (unwired) "查询系统状态" ("当前解析模式")
            n152 = call "超标留样通讯.vi"("error in (no error)"=w245, "功能输入"=enum16{"打开串口", "写入", "读取", "关闭串口"}."读取") -> ("error out"=w238:errorcluster, "读取缓冲区"=w241:string)  [unwired: 7 in, 1 out]
            "读取缓冲区" <- w241
            n153 = case shown="\"查询瓶记录\"" w236 {
              tunnel: w241 -> [w246 w254 w262 w270 w278 w285 w291 w297 w304]
              frame "触发采样" {
                n154 = flat-sequence {
                  tunnel: w246 -> [w247]
                  frame #0 {
                    n155 = disable-structure shown="禁用" {
                      disable-tunnel: w247 -> [w251 _]
                      frame Disabled {
                        n156 = Equal?(x=w251, y="ÌÝªð»") -> (x = y?=w249:bool)
                        n157 = case shown="真" w249 {
                          tunnel: ["触发采样失败！" ("消息") "触发采样成功！" ("消息")] -> w248
                          frame False {
                          }
                          frame True {
                          }
                        }
                        n158 = One Button Dialog(message=w248) -> ()  [unwired: 1 in, 1 out]
                      }
                      frame Enabled {
                      }
                    }
                  }
                }
              }
              frame "供样命令" {
                n159 = flat-sequence {
                  tunnel: w254 -> [w255]
                  frame #0 {
                    n160 = disable-structure shown="禁用" {
                      disable-tunnel: w255 -> [w259 _]
                      frame Disabled {
                        n161 = Equal?(x=w259, y="ÌÝª\u0010»") -> (x = y?=w257:bool)
                        n162 = case shown="真" w257 {
                          tunnel: ["供样失败！" ("消息") "供样成功！" ("消息")] -> w256
                          frame False {
                          }
                          frame True {
                          }
                        }
                        n163 = One Button Dialog(message=w256) -> ()  [unwired: 1 in, 1 out]
                      }
                      frame Enabled {
                      }
                    }
                  }
                }
              }
              frame "留样命令", Default {
                n164 = flat-sequence {
                  tunnel: w262 -> [w263]
                  frame #0 {
                    n165 = disable-structure shown="禁用" {
                      disable-tunnel: w263 -> [w267 _]
                      frame Disabled {
                        n166 = Equal?(x=w267, y="ÌÝª\u0011»") -> (x = y?=w265:bool)
                        n167 = case shown="真" w265 {
                          tunnel: ["留样失败！" ("消息") "留样成功！" ("消息")] -> w264
                          frame False {
                          }
                          frame True {
                          }
                        }
                        n168 = One Button Dialog(message=w264) -> ()  [unwired: 1 in, 1 out]
                      }
                      frame Enabled {
                      }
                    }
                  }
                }
              }
              frame "复位指令" {
                n169 = flat-sequence {
                  tunnel: w270 -> [w271]
                  frame #0 {
                    n170 = disable-structure shown="禁用" {
                      disable-tunnel: w271 -> [w275 _]
                      frame Disabled {
                        n171 = Equal?(x=w275, y="ÌÝª2»") -> (x = y?=w273:bool)
                        n172 = case shown="真" w273 {
                          tunnel: ["复位失败！" ("消息") "复位成功！" ("消息")] -> w272
                          frame False {
                          }
                          frame True {
                          }
                        }
                        n173 = One Button Dialog(message=w272) -> ()  [unwired: 1 in, 1 out]
                      }
                      frame Enabled {
                      }
                    }
                  }
                }
              }
              frame "远程取样" {
                n174 = flat-sequence {
                  tunnel: w278 -> [w282]
                  frame #0 {
                    n175 = Equal?(x=w282, y="ÌÝª3»") -> (x = y?=w280:bool)
                    n176 = case shown="假" w280 {
                      tunnel: ["远程取样失败！" ("消息") "远程取样成功！" ("消息")] -> w279
                      frame False {
                      }
                      frame True {
                      }
                    }
                    n177 = One Button Dialog(message=w279) -> ()  [unwired: 1 in, 1 out]
                  }
                }
              }
              frame "查询采样记录" {
                n178 = flat-sequence {
                  tunnel: w285 -> [w290]
                  frame #0 {
                    n179 = call "科盛查询命令解析.vi"("解析参数选择"=enum16{"查询采样记录", "查询瓶记录", "查询系统状态"}."查询采样记录", "命令输入"=w290) -> ("Variant"=w288:variant)  [unwired: 9 in]
                    n180 = Variant To Data(type=T15 [] ("输出数组"), Variant=w288) -> (data=w286:T15)  [unwired: 1 in, 1 out]
                    n181 = global write "超标留样全局.vi" "查询采样记录"(w286) -> ()
                  }
                }
              }
              frame "查询瓶记录" {
                n182 = flat-sequence {
                  tunnel: w291 -> [w296]
                  frame #0 {
                    n183 = call "科盛查询命令解析.vi"("解析参数选择"=enum16{"查询采样记录", "查询瓶记录", "查询系统状态"}."查询瓶记录", "命令输入"=w296) -> ("Variant"=w294:variant)  [unwired: 9 in]
                    n184 = Variant To Data(type=T16 {"瓶1采样量(ml)"=0.0, "瓶2采样量(ml)"=0.0, "瓶3采样量(ml)"=0.0, "瓶4采样量(ml)"=0.0, "瓶5采样量(ml)"=0.0, "瓶6采样量(ml)"=0.0, "瓶7采样量(ml)"=0.0, "瓶8采样量(ml)"=0.0, "瓶9采样量(ml)"=0.0, "瓶10采样量(ml)"=0.0, "瓶11采样量(ml)"=0.0, "瓶12采样量(ml)"=0.0, "瓶13采样量(ml)"=0.0, "瓶14采样量(ml)"=0.0, "瓶15采样量(ml)"=0.0, "瓶16采样量(ml)"=0.0, "瓶17采样量(ml)"=0.0, "瓶18采样量(ml)"=0.0, "瓶19采样量(ml)"=0.0, "瓶20采样量(ml)"=0.0, "瓶21采样量(ml)"=0.0, "瓶22采样量(ml)"=0.0, "瓶23采样量(ml)"=0.0, "瓶24采样量(ml)"=0.0} ("查询瓶记录"), Variant=w294) -> (data=w292:T16)  [unwired: 1 in, 1 out]
                    n185 = global write "超标留样全局.vi" "查询瓶记录"(w292) -> ()
                  }
                }
              }
              frame "清除瓶记录" {
                n186 = flat-sequence {
                  tunnel: w297 -> [w301]
                  frame #0 {
                    n187 = Equal?(x=w301, y="ÌÝª1»") -> (x = y?=w299:bool)
                    n188 = case shown="假" w299 {
                      tunnel: ["清除失败！" ("消息") "清除成功！" ("消息")] -> w298
                      frame False {
                      }
                      frame True {
                      }
                    }
                    n189 = One Button Dialog(message=w298) -> ()  [unwired: 1 in, 1 out]
                  }
                }
              }
              frame "查询系统状态" {
                n190 = flat-sequence {
                  tunnel: w304 -> [w305]
                  frame #0 {
                    n191 = case shown="\"假\", 默认" w305 {
                      tunnel: w305 -> [w308 _]
                      frame "假", Default {
                        n192 = call "科盛查询命令解析.vi"("解析参数选择"=enum16{"查询采样记录", "查询瓶记录", "查询系统状态"}."查询系统状态", "命令输入"=w308) -> ("Variant"=w310:variant)  [unwired: 9 in]
                        n193 = Variant To Data(type=T5 {"采样模式"=enum."定时定量1", "仪器状态"=enum."待机", "仪器时间"="", "瞬时流速(m3/s)"=0.0, "当前COD值(mg/L)"=0.0, "当前氨氮值(mg/L)"=0.0, "当前温度(℃)"=0.0, "开关量状态1"="", "开关量状态2"="", "开关量状态3"="", "A桶水样量(mL)"=0.0, "B桶水样量(mL)"=0.0} ("查询系统状态"), Variant=w310) -> (data=w307:T5)  [unwired: 1 in, 1 out]
                        "查询系统状态" <- w307
                        n194 = global write "超标留样全局.vi" "查询系统状态"(w307) -> ()
                      }
                      frame "" {
                      }
                    }
                    n195 = Equal?(x=w305, y="ÌÝª\u0001»") -> ()  [unwired: 1 out]
                  }
                }
              }
            }
            n196 = Unbundle By Name(w238) -> ("status"=w240:bool, "source"=→"source":string)
            n197 = Not(x=w240) -> (.not. x?=w237:bool)
            "通讯" <- w237
            n198 = global write "超标留样全局.vi" "通讯"(w237) -> ()
          }
          frame "write" {
            n199 = call "超标留样通讯.vi"("error in (no error)"=w319, "写入缓冲区"=w316, "功能输入"=enum16{"打开串口", "写入", "读取", "关闭串口"}."写入") -> ("error out"=w317:errorcluster)  [unwired: 6 in, 2 out]
            n200 = Bundle By Name(cluster=w315, "枚举"=enum16{"open", "read", "write", "close"}."read" ("元素"), "解析字符串"=w313) -> (w312:T6)
            n201 = Enqueue Element(queue=w323, element=w312, error in (no error)=w322) -> (queue out=w321:refnum<queue>, error out=w320:errorcluster)  [unwired: 1 in, 1 out]
          }
          frame "close" {
            n202 = call "超标留样通讯.vi"("error in (no error)"=w333, "功能输入"=enum16{"打开串口", "写入", "读取", "关闭串口"}."关闭串口") -> ("error out"=w331:errorcluster)  [unwired: 7 in, 2 out]
            n203 = Bundle By Name(cluster=T6 {"枚举"=enum."open", "写入字符串"="", "解析字符串"=""}, "枚举"=enum16{"open", "read", "write", "close"}."open" ("元素")) -> (w324:T6)
            n204 = Enqueue Element(queue=w330, element=w324, error in (no error)=w329) -> (queue out=w328:refnum<queue>, error out=w327:errorcluster)  [unwired: 1 in, 1 out]
          }
        }
      }
      frame Error {
        n205 = Flush Queue(queue=w345, error in (no error)=w344) -> (queue out=w343:refnum<queue>, error out=w342:errorcluster)  [unwired: 1 out]
        n206 = call <vilib>:"Clear Errors.vi"("error in (no error)"=w341) -> ("error out"=w340:errorcluster)  [unwired: 5 in, 1 out]
        n207 = Wait (ms)(milliseconds to wait=u32 2000 ("等待时间（毫秒）")) -> ()  [unwired: 1 out]
        n208 = Bundle By Name(cluster=T6 {"枚举"=enum."open", "写入字符串"="", "解析字符串"=""}, "枚举"=enum16{"open", "read", "write", "close"}."close" ("元素")) -> (w334:T6)
        n209 = Enqueue Element(queue=w343, element=w334, error in (no error)=w342) -> (queue out=w339:refnum<queue>, error out=w338:errorcluster)  [unwired: 1 in, 1 out]
      }
    }
  }
  n210 = Close Reference(reference=w4, error in (no error)=w3) -> ()  [unwired: 1 out]
  n211 = Obtain Queue(name (unnamed)="超标留样外部交互" ("名称（未命名）"), element data type=T7 {"STEP"=enum."write", "写入缓冲区"="ª\u0006\u0000\u0000P`\u00000»"}) -> (queue out=w11:refnum<queue>, error out=w10:errorcluster)  [unwired: 3 in, 1 out]
  n212 = while {
    tunnel: w11 -> [w352]
    tunnel: w10 -> [w351]
    tunnel: [w346] -> _
    stop <- FALSE stop-if-true
    n213 = Dequeue Element(queue=w352, error in (no error)=w351) -> (element=w350:T7, error out=w348:errorcluster)  [unwired: 1 in, 2 out]
    n214 = Unbundle By Name(w350) -> ("STEP"=w349:enum16{"open", "read", "write", "close"}, "写入缓冲区"=w347:string)
    n215 = case shown="\"write\"" w349 {
      tunnel: w348 -> [_ w354 w358 _]
      tunnel: w347 -> [_ _ w357 _]
      tunnel: [_ _ w356 _] -> w346
      frame "open", Default {
      }
      frame "read" {
        n216 = call "超标留样通讯.vi"("error in (no error)"=w354, "功能输入"=enum16{"打开串口", "写入", "读取", "关闭串口"}."读取") -> ()  [unwired: 7 in, 3 out]
      }
      frame "write" {
        n217 = call "超标留样通讯.vi"("error in (no error)"=w358, "写入缓冲区"=w357, "功能输入"=enum16{"打开串口", "写入", "读取", "关闭串口"}."写入") -> ("error out"=w356:errorcluster)  [unwired: 6 in, 2 out]
      }
      frame "close" {
      }
    }
  }
